vi "ReadData.vi"(8 "error in (no error)":errorcluster, 11 "object in":refnum<class "Modbus.lvclass">) -> (0 "error out":errorcluster, 2 "read buffer":string, 3 "object out":refnum<class "Modbus.lvclass">)   [LabVIEW 2019, in "Modbus.lvclass"]
uses:
  Modbus.lvclass
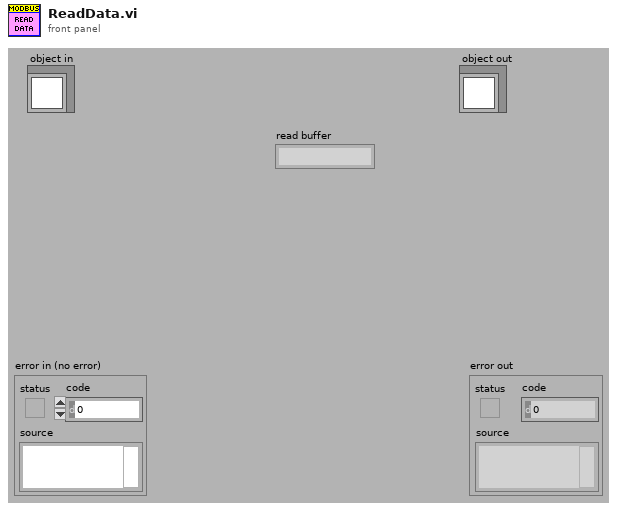
[diagram p1: front panel]
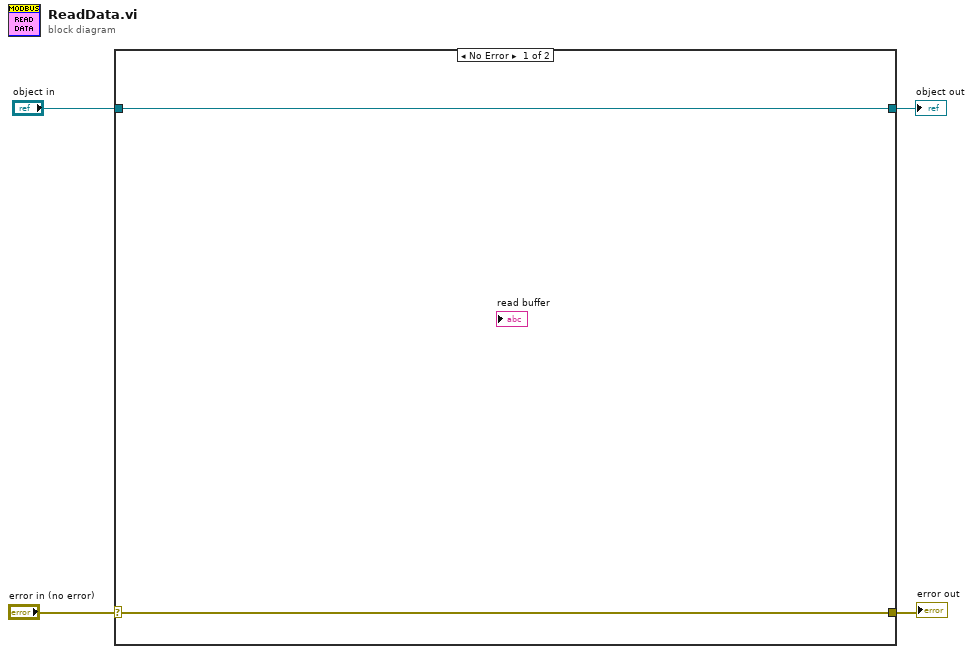
[diagram p0: block diagram]
diagram:
  n1 = case shown="No Error" "error in (no error)" {
    selector: "error in (no error)" -> [w6 w8]
    tunnel: [w6 w8] -> w3
    tunnel: [w5 w7] -> w1
    tunnel: "object in" -> [w5 w7]
    frame No Error {
    }
    frame Error {
    }
  }
  "error out" <- w3
  "object out" <- w1
